vi "Unflatten Buffer Configuration.vi"(11 "Flattened Configuration":u8[](array[numeric]) format="%.0x") -> (3 "Buffer Configuration":T1)   [LabVIEW 2021, in "CIF_CIPC_Chn.lvclass"]
uses:
  CIF_CIPC_Chn.lvclass
  Typedef/Buffer Configuration Data.ctl
  CIF_CIPC_Chn.lvclass/CIF_CIPC_Chn.ctl
  <vilib>/CIF Foundation/CIF Utilities/DataTypes/DataTypes_CIF_U.lvlib
  <vilib>/CIF Foundation/CIF CIPC/TypeDefs/Backpressure References.ctl
  <vilib>/CIF Foundation/CIF CIPC/CIF_NI_CIPC.lvlib
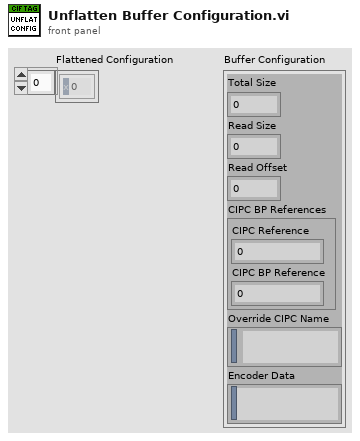
[diagram p1: front panel]
types:
  T1 = typedef "CIF_CIPC_Chn.lvclass/Buffer Configuration Data.ctl" = cluster{"Total Size":u32, "Read Size":u32, "Read Offset":u32, "CIPC BP References":T2, "Override CIPC Name":string, "Encoder Data":string}
  T2 = typedef "CIF_NI_CIPC.lvlib/Backpressure References.ctl" = cluster{"CIPC Reference":u64, "CIPC BP Reference":u64}
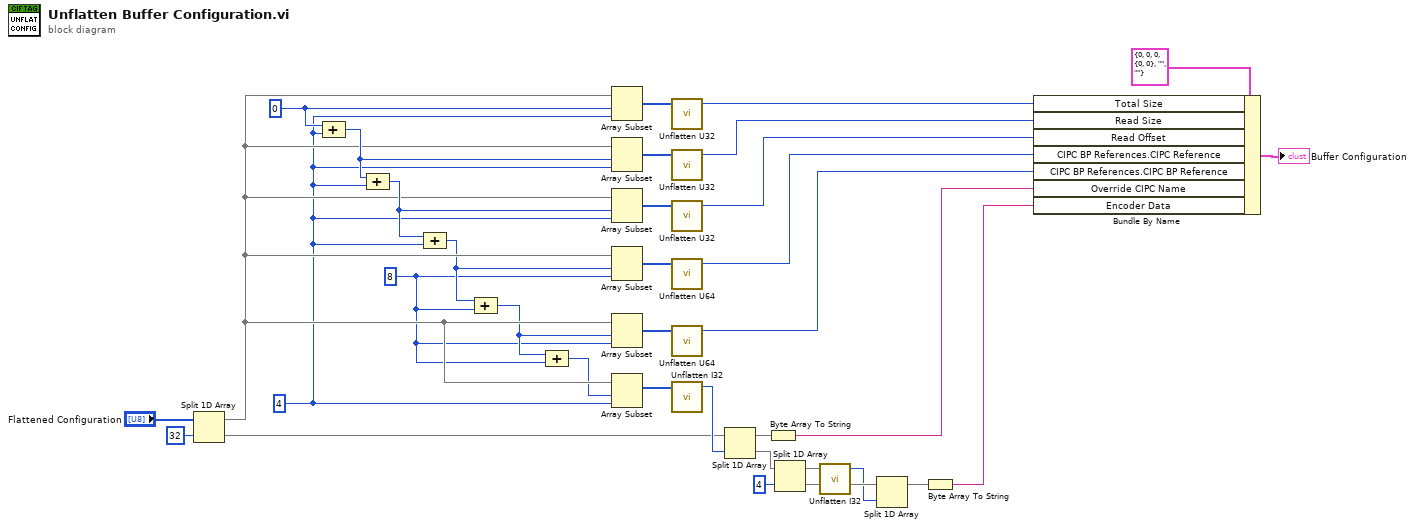
[diagram p0: block diagram]
diagram:
  w1 = 8 ("length")
  w5 = 4 ("length")
  w33 = 0 ("index")
  n1 = Split 1D Array(array="Flattened Configuration", index=32) -> (first subarray=w9:u8[], second subarray=w21:u8[])
  n2 = Compound Arithmetic op=unknown(w33, w5) -> (w32:i32)
  n3 = Compound Arithmetic op=unknown(w32, w5) -> (w23:i32)
  n4 = Compound Arithmetic op=unknown(w23, w5) -> (w8:i32)
  n5 = Compound Arithmetic op=unknown(w8, w1) -> (w7:i32)
  n6 = Compound Arithmetic op=unknown(w7, w1) -> (w6:i32)
  n7 = Array Subset(array=w9, index=w33, length=w5) -> (w29:u8[])
  n8 = Array Subset(array=w9, index=w32, length=w5) -> (w30:u8[])
  n9 = Array Subset(array=w9, index=w23, length=w5) -> (w31:u8[])
  n10 = Array Subset(array=w9, index=w8, length=w1) -> (w11:u8[])
  n11 = Array Subset(array=w9, index=w7, length=w1) -> (w10:u8[])
  n12 = Array Subset(array=w9, index=w6, length=w5) -> (w4:u8[])
  n13 = call <vilib>:"Unflatten U32.vi"("Flat Data"=w29) -> ("U32"=w28:u32)  [unwired: 4 in]
  n14 = call <vilib>:"Unflatten U32.vi"("Flat Data"=w30) -> ("U32"=w27:u32)  [unwired: 4 in]
  n15 = call <vilib>:"Unflatten U32.vi"("Flat Data"=w31) -> ("U32"=w26:u32)  [unwired: 4 in]
  n16 = call <vilib>:"Unflatten U64.vi"("Flat Data"=w11) -> ("U64"=w3:u64)  [unwired: 4 in]
  n17 = call <vilib>:"Unflatten U64.vi"("Flat Data"=w10) -> ("U64"=w2:u64)  [unwired: 4 in]
  n18 = call <vilib>:"Unflatten I32.vi"("Flat Data"=w4) -> ("I32"=w22:i32)  [unwired: 4 in]
  n19 = Split 1D Array(array=w21, index=w22) -> (first subarray=w20:u8[], second subarray=w18:u8[])
  n20 = Byte Array To String(unsigned byte array=w20) -> (string=w19:string)
  n21 = Split 1D Array(array=w18, index=4) -> (first subarray=w15:u8[], second subarray=w14:u8[])
  n22 = call <vilib>:"Unflatten I32.vi"("Flat Data"=w15) -> ("I32"=w13:i32)  [unwired: 4 in]
  n23 = Split 1D Array(array=w14, index=w13) -> (first subarray=w12:u8[])  [unwired: 1 out]
  n24 = Byte Array To String(unsigned byte array=w12) -> (string=w16:string)
  n25 = Bundle By Name(cluster=T1 {"Total Size"=0, "Read Size"=0, "Read Offset"=0, "CIPC BP References"={"CIPC Reference"=0, "CIPC BP Reference"=0}, "Override CIPC Name"="", "Encoder Data"=""} ("Buffer Configuration"), "Total Size"=w28, "Read Size"=w27, "Read Offset"=w26, "CIPC BP References.CIPC Reference"=w3, "CIPC BP References.CIPC BP Reference"=w2, "Override CIPC Name"=w19, "Encoder Data"=w16) -> (→"Buffer Configuration":T1)
